vi "OAT Tachless Get Order Profile at Cursor.vi"(10 "Cursor Position":cluster{"Cursor X":dbl, "Cursor Y":dbl} {"Cursor Y" format="%.2f"; "Cursor X" format="%.2f"}, 11 "speed profile":T1 {"speed [RPM]" format="%.2f"; "time [s]" format="%.2f"}) -> (1 "order at cursor":dbl format="%.2f", 3 "Profile at Cursor":cluster{"time [s]":dbl[], dbl[]} {"?" format="%.2f"; "time [s]" format="%.2f"})   [LabVIEW 2017, in "SoundVib_Tachless.lvlib"]
uses:
  <vilib>/addons/Sound and Vibration/Order Analysis/Tachless/SoundVib_Tachless.lvlib
  <vilib>/addons/Sound and Vibration/Order Analysis/Tach Process/SubVIs/speed profile.ctl
  <vilib>/addons/Sound and Vibration/Order Analysis/Tach Process/SoundVib_TachProcess.lvlib
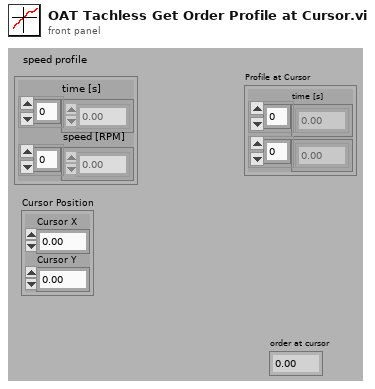
[diagram p1: front panel]
types:
  T1 = typedef "SoundVib_TachProcess.lvlib/speed profile.ctl" = cluster{"time [s]":dbl[], "speed [RPM]":dbl[]}
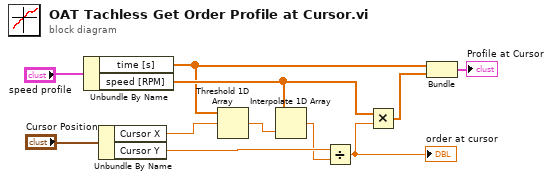
[diagram p0: block diagram]
diagram:
  n1 = Unbundle By Name("speed profile") -> ("time [s]"=w4:dbl[], "speed [RPM]"=w5:dbl[])
  n2 = Unbundle By Name("Cursor Position") -> ("Cursor X"=w9:dbl, "Cursor Y"=w7:dbl)
  n3 = Threshold 1D Array(2:w9, 3:w4) -> (0:w8:dbl)  [unwired: 1 in]
  n4 = Interpolate 1D Array(1:w8, 2:w5) -> (0:w6:dbl)
  n5 = Divide(x=w7, y=w6) -> (x/y=w1:dbl)
  "order at cursor" <- w1
  n6 = Multiply(x=w5, y=w1) -> (x*y=w3:dbl[])
  n7 = Bundle("time [s]"=w4, w3) -> (→"Profile at Cursor":cluster{"time [s]":dbl[], dbl[]})  [unwired: 1 in]
